vi "Test Refresh Returned Amounts.vi"(8 "error in (no error)":errorcluster) -> (0 "error out":errorcluster)   [LabVIEW 2019]
uses:
  Setting Database/Setting Database.lvclass
  C:/Program Files (x86)/National Instruments/LabVIEW 2019/vi.lib/JKI/JKI SMO/SMO/SMO.lvclass
  Setting Database/Typedefs/PrivateEvents--Setting Database.Refresh.ctl
  Path Settings/Path Settings.lvclass
  C:/Users/Albro/Documents/GitHub/AFM-Lithography/lvsrc/Classes/Settings/ObjectSettings/ObjectSettings.lvclass
  Dot Settings/Dot Settings.lvclass
  Rectangle Settings/Rectangle Settings.lvclass
  Funnel Settings/Funnel Settings.lvclass
  <vilib>/addons/_JKI Toolkits/Caraya/classes/Assert/Assert Equal Value_Variant.vi
  <vilib>/addons/_JKI Toolkits/Caraya/classes/Test/Test.lvclass
  <vilib>/addons/_JKI Toolkits/Caraya/classes/Assert/Assert.lvclass
  <vilib>/JKI/JKI SMO/SMO/SMO.lvclass
  <vilib>/LabVIEW Open Source Project/Unicity/RandomStringGenerator/RandomStringGenerator.lvclass
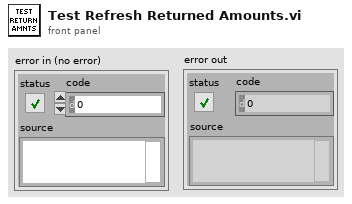
[diagram p1: front panel]
types:
  T1 = typedef "Setting Database.lvclass/PrivateEvents--Setting Database.Refresh.ctl" = cluster{"Paths":string[], "Rectangles":string[], "Funnels":string[], "Dots":string[]}
  T2 = typedef "Setting Database.lvclass/PublicEvents--Cluster.ctl" = cluster{"NewActivePath":refnum<user-event>, "PathsUpdated":refnum<user-event>, "RectanglesUpdated":refnum<user-event>, "NewActiveRectangle":refnum<user-event>, "NewActiveFunnel":refnum<user-event>, "FunnelsUpdated":refnum<user-event>, "NewActiveDot":refnum<user-event>, "DotsUpdated":refnum<user-event>}
  T3 = typedef "Setting Database.lvclass/PublicEvents--Setting Database.PathsUpdated.ctl" = refnum<class "Path Settings.lvclass">[]
  T4 = typedef "Setting Database.lvclass/PublicEvents--Setting Database.DotsUpdated.ctl" = refnum<class "Dot Settings.lvclass">[]
  T5 = typedef "Setting Database.lvclass/PublicEvents--Setting Database.RectanglesUpdated.ctl" = refnum<class "Rectangle Settings.lvclass">[]
  T6 = typedef "Setting Database.lvclass/PublicEvents--Setting Database.FunnelsUpdated.ctl" = refnum<class "Funnel Settings.lvclass">[]
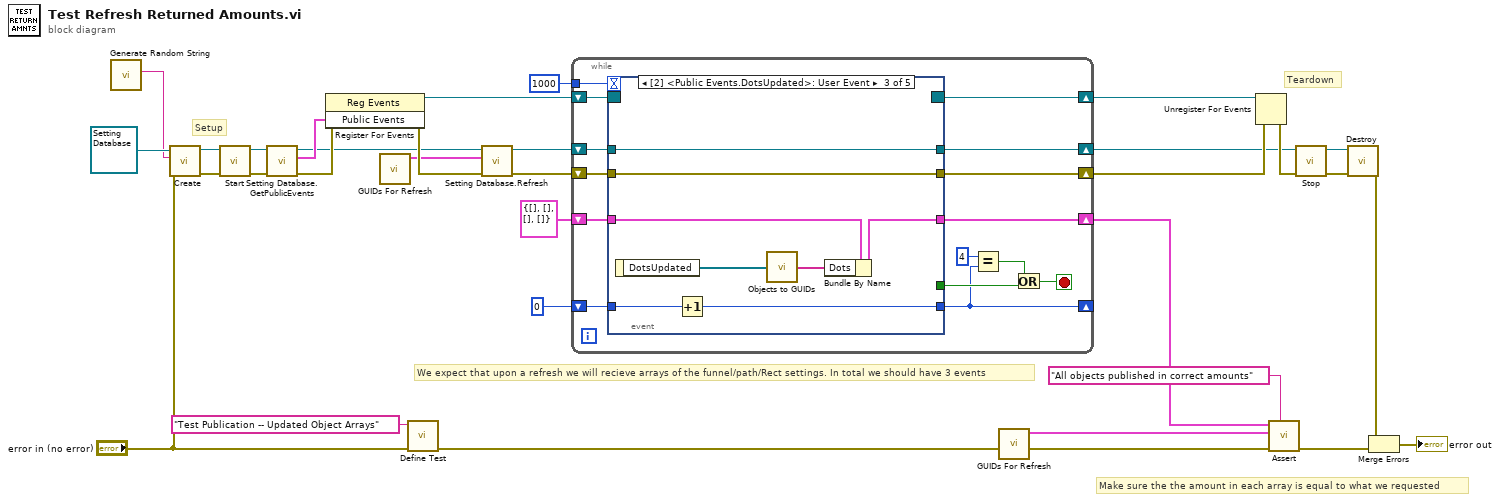
[diagram p0: block diagram]
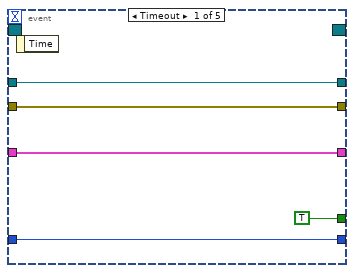
[diagram p2: hidden frame]
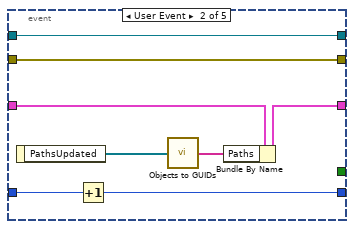
[diagram p3: hidden frame]
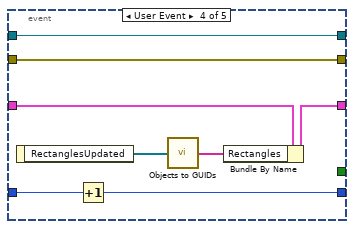
[diagram p4: hidden frame]
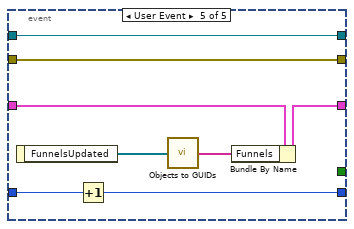
[diagram p5: hidden frame]
diagram:
  # "Make sure the the amount in each array is equal to what we requested"
  # "We expect that upon a refresh we will recieve arrays of the funnel/path/Rect settings. In total we should have 3 events"
  # "Teardown"
  # "Setup"
  n1 = call <vilib>:"Generate Random String.vi"() -> ("Random String"=w1:string)  [unwired: 11 in]
  n2 = call <vilib>:"Create.vi"("error in (no error)"="error in (no error)", "Subsystem Name (optional)"=w1, "SMO"=refnum<class "Setting Database.lvclass"> refnum ("Setting Database.lvclass")) -> ("error out"=w29:errorcluster, "SMO out"=w20:refnum<class "Setting Database.lvclass">)  [unwired: 6 in, 1 out]
  n3 = call <vilib>:"Start.vi"("error in (no error)"=w29, "SMO"=w20) -> ("error out"=w28:errorcluster, "SMO out"=w19:refnum<class "Setting Database.lvclass">)  [unwired: 8 in]
  n4 = call "Setting Database.GetPublicEvents.vi"("error in (no error)"=w28, "Setting Database"=w19) -> ("error out"=w24:errorcluster, "Public Events"=w14:T2, "Setting Database out"=w11:refnum<class "Setting Database.lvclass">)  [unwired: 7 in]
  n5 = register-events(error in=w24, w14) -> (reference out=w16:refnum<event-registration>, error out=w12:errorcluster)  [unwired: 1 in]
  n6 = call "GUIDs For Refresh.vi"() -> ("Initialize"=w3:T1)  [unwired: 11 in]
  n7 = call <vilib>:"Define Test.vi"("error in (no error)"="error in (no error)", "Label (VI Title)"="Test Publication -- Updated Object Arrays") -> ("error out"=w31:errorcluster)  [unwired: 8 in, 1 out]
  n8 = call "Setting Database.Refresh.vi"("error in (no error)"=w12, "Initialize"=w3, "Setting Database"=w11) -> ("error out"=w9:errorcluster, "Setting Database out"=w10:refnum<class "Setting Database.lvclass">)  [unwired: 7 in]
  n9 = while {
    shift-right: [w46] -> w17
    shift-left: w16 -> [w45]
    shift-right: [w44] -> w15
    shift-left: w10 -> [w43]
    shift-right: [w47] -> w26
    shift-left: w9 -> [w42]
    shift-right: [w33] -> _
    shift-left: 0 -> [w41]
    tunnel: 1000 -> [w39]
    shift-right: [w38] -> w5
    shift-left: T1 {"Paths"=[], "Rectangles"=[], "Funnels"=[], "Dots"=[]} ("Initialize") -> [w40]
    stop <- w35 stop-if-true
    n10 = event shown="[2] <Public Events.DotsUpdated>: User Event" {
      selector: w45 -> [_ _ _ _ _]
      dyn-events: [_ _ _ _ _] -> w46
      timeout: w39 -> [_ _ _ _ _]
      tunnel: [w52 w60 w68 w76 w84] -> w47
      tunnel: w42 -> [w52 w60 w68 w76 w84]
      tunnel: w43 -> [w51 w59 w67 w75 w83]
      tunnel: [w51 w59 w67 w75 w83] -> w44
      tunnel: w41 -> [w50 w58 w66 w74 w82]
      tunnel: [w50 w57 w65 w73 w81] -> w33
      tunnel: w40 -> [w48 w56 w64 w72 w80]
      tunnel: [w48 w55 w63 w71 w79] -> w38
      tunnel: [TRUE _ _ _ _] -> w34
      event Timeout {
        n11 = event-data() -> ()  [unwired: 1 in, 1 out]
      }
      event User Event {
        n12 = event-data() -> ("PathsUpdated"=w54:T3)  [unwired: 1 in]
        n13 = Increment(x=w58) -> (x+1=w57:i32)
        n14 = call "Objects to GUIDs.vi"("Objects"=w54) -> ("GUIDs"=w53:string[])  [unwired: 3 in, 1 out]
        n15 = Bundle By Name(cluster=w56, "Paths"=w53) -> (w55:T1)
      }
      event User Event {
        n16 = event-data() -> ("DotsUpdated"=w62:T4)  [unwired: 1 in]
        n17 = Increment(x=w66) -> (x+1=w65:i32)
        n18 = call "Objects to GUIDs.vi"("Objects"=w62) -> ("GUIDs"=w61:string[])  [unwired: 3 in, 1 out]
        n19 = Bundle By Name(cluster=w64, "Dots"=w61) -> (w63:T1)
      }
      event User Event {
        n20 = event-data() -> ("RectanglesUpdated"=w70:T5)  [unwired: 1 in]
        n21 = Increment(x=w74) -> (x+1=w73:i32)
        n22 = call "Objects to GUIDs.vi"("Objects"=w70) -> ("GUIDs"=w69:string[])  [unwired: 3 in, 1 out]
        n23 = Bundle By Name(cluster=w72, "Rectangles"=w69) -> (w71:T1)
      }
      event User Event {
        n24 = event-data() -> ("FunnelsUpdated"=w78:T6)  [unwired: 1 in]
        n25 = Increment(x=w82) -> (x+1=w81:i32)
        n26 = call "Objects to GUIDs.vi"("Objects"=w78) -> ("GUIDs"=w77:string[])  [unwired: 3 in, 1 out]
        n27 = Bundle By Name(cluster=w80, "Funnels"=w77) -> (w79:T1)
      }
    }
    n28 = Equal?(x=4, y=w33) -> (x = y?=w36:bool)
    n29 = Or(x=w36, y=w34) -> (x .or. y?=w35:bool)
  }
  n30 = call "GUIDs For Refresh.vi"() -> ("Initialize"=w2:T1)  [unwired: 11 in]
  n31 = Unregister For Events(event registration refnum=w17, error in=w26) -> (error out=w25:errorcluster)
  n32 = call-poly <vilib>:"Assert.vi"("Label"="All objects published in correct amounts" ("Label (VI Title)"), "error in (no error)"=w31, "Actual"=w2, "Expected"=w5) -> ("error out"=w32:errorcluster)  [unwired: 6 in, 1 out]
  n33 = call <vilib>:"Stop.vi"("error in (no error)"=w25, "SMO"=w15) -> ("error out"=w27:errorcluster, "SMO out"=w18:refnum<class "Setting Database.lvclass">)  [unwired: 8 in]
  n34 = call <vilib>:"Destroy.vi"("error in (no error)"=w27, "SMO"=w18) -> ("error out"=w23:errorcluster)  [unwired: 9 in]
  n35 = Merge Errors(w23, w32) -> (→"error out":errorcluster)
